vi "Pre Launch Init.vi"(11 "Broadcast Actor in":refnum<class "Broadcast Actor.lvclass">) -> (0 "error out":errorcluster, 3 "Broadcast Actor out":refnum<class "Broadcast Actor.lvclass">)   [LabVIEW 2017, in "Broadcast Actor.lvlib" / "Broadcast Actor.lvclass"]
doc: "(<B>Filename</B>: Actor Framework.lvlib:Actor.lvclass:Pre Launch Init.vi)\n\nDefines behavior that occurs after the Launch Nested Actor method is invoked but before the actor's Actor Core method begins running.\n\nBy default, this method does nothing. A descendant class may override it to define behavior."
uses:
  Broadcast Actor.lvclass
  Broadcast Actor.lvclass/Broadcast Actor.ctl
  <vilib>/ActorFramework/Actor/Actor.lvclass
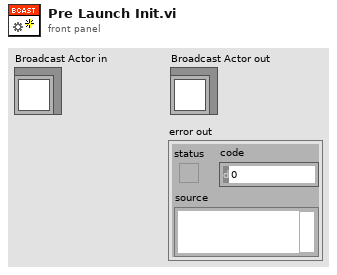
[diagram p1: front panel]
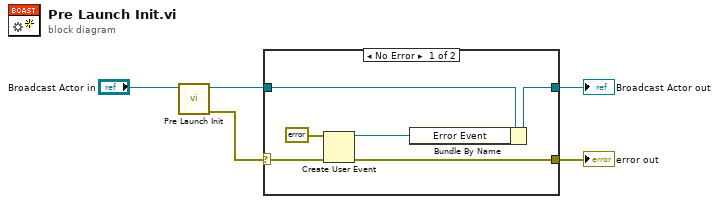
[diagram p0: block diagram]
diagram:
  n1 = call-parent "Pre Launch Init.vi"("Actor in"="Broadcast Actor in") -> ("error out"=w1:errorcluster, "Actor out"=w5:refnum<class "Broadcast Actor.lvclass">)  [unwired: 9 in]
  n2 = case shown="No Error" w1 {
    selector: w1 -> [w6 w12]
    tunnel: w5 -> [w11 w13]
    tunnel: [w10 w13] -> w3
    tunnel: [w9 w12] -> w2
    frame No Error {
      n3 = Create User Event(user event datatype=errorcluster {"status"=FALSE, "code"=0, "source"=""} ("error in (no error)"), error in=w6) -> (user event=w7:refnum<user-event>, error out=w9:errorcluster)
      n4 = Bundle By Name(cluster=w11, "Error Event"=w7) -> (w10:refnum<class "Broadcast Actor.lvclass">)
    }
    frame Error {
    }
  }
  "error out" <- w2
  "Broadcast Actor out" <- w3
